vi "plot-realtime-sub0.vi"(1 "索引":i32, 2 "x":dbl) -> (0 "数组":dbl[](array[numeric]))   [LabVIEW 2014]
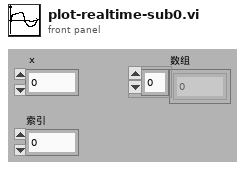
[diagram p1: front panel]
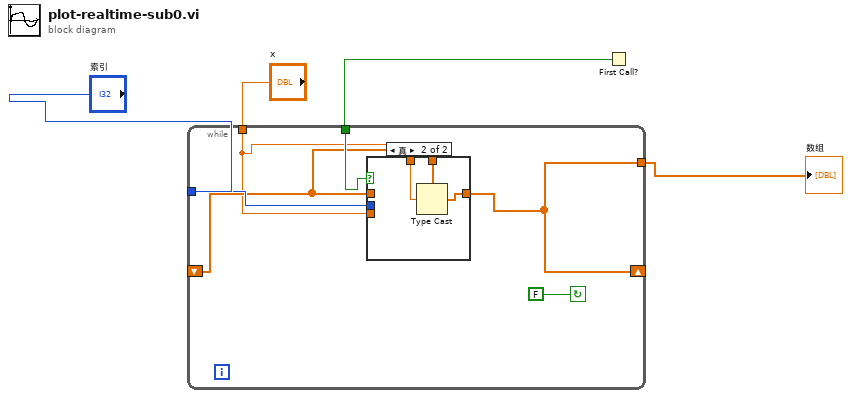
[diagram p0: block diagram]
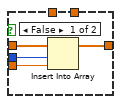
[diagram p2: hidden frame]
diagram:
  n1 = First Call?() -> (First Call?: T/F=w1:bool)
  n2 = while {
    tunnel: "索引" -> [w10]
    tunnel: "x" -> [w5]
    tunnel: [w8] -> w2
    shift-right: [w8] -> _
    shift-left: _ -> [w6]
    tunnel: w1 -> [w7]
    stop <- FALSE continue-if-true
    n3 = case shown="真" w7 {
      tunnel: w10 -> [w13 _]
      tunnel: w5 -> [w12 _]
      tunnel: w6 -> [w14 _]
      tunnel: [w11 w17] -> w8
      tunnel: w6 -> [_ w16]
      tunnel: w5 -> [_ w15]
      frame False {
        n4 = Insert Into Array(array=w14, index=w13, new element=w12) -> (w11:dbl[])
      }
      frame True {
        n5 = Type Cast(type=w16, x=w15) -> (*(type *) &x=w17:dbl[])
      }
    }
  }
  "数组" <- w2
